vi "Send command Get Pin.vi"(7 "Marca":string, 8 "error in (no error)":errorcluster, 9 "Pin":string, 10 "Puerto":string, 11 "Simulado in":refnum<class "Simulado.lvclass">) -> (0 "error out":errorcluster, 1 "Command":string, 2 "Expected response":string, 3 "Simulado out":refnum<class "Simulado.lvclass">)   [LabVIEW 2020, in "Simulado.lvclass"]
uses:
  Simulado.lvclass
  D:/Fork/IVProyecto_3P/Abstract/Serial Device/Serial Device.lvclass
  Abstract/Serial Device/Serial Device.lvclass
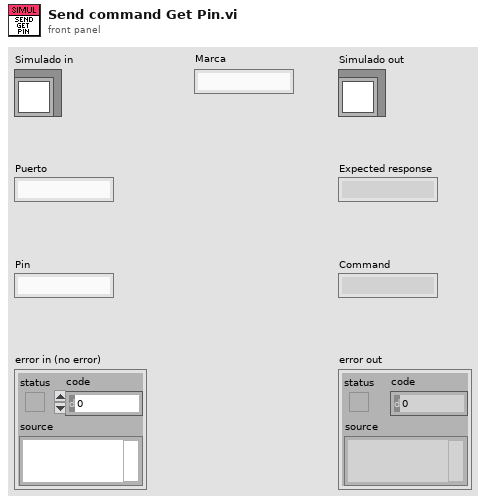
[diagram p1: front panel]
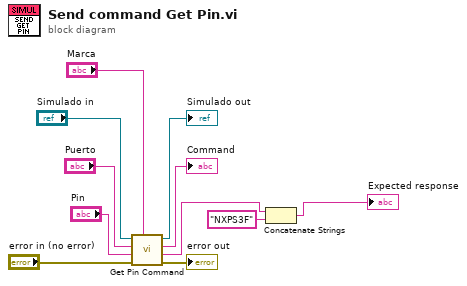
[diagram p0: block diagram]
diagram:
  n1 = call "Get Pin Command.vi"("Marca"="Marca", "error in (no error)"="error in (no error)", "Pin"="Pin", "Puerto"="Puerto", "Serial Device in"="Simulado in") -> ("error out"=→"error out":errorcluster, "Expected response"=w3:string, "Command"=→"Command":string, "Serial Device out"=→"Simulado out":refnum<class "Simulado.lvclass">)  [unwired: 3 in]
  n2 = Concatenate Strings(w3, "NXPS3F" ("string")) -> (→"Expected response":string)
